vi "Vision 1.vi"(6 "Blue":cluster{"Lower value":i32, "Upper value":i32}={"Lower value"=0, "Upper value"=20}, 8 "Green":cluster{"Lower value":i32, "Upper value":i32}={"Lower value"=0, "Upper value"=20}, 10 "Red":cluster{"Lower value":i32, "Upper value":i32}={"Lower value"=0, "Upper value"=20}, 11 "RGB":T1) -> (0 "RGB":T1, 4 "Binary":T1)   [LabVIEW 2014]
uses:
  <vilib>/vision/Image Controls.llb/IMAQ Image.ctl
  <vilib>/vision/NI_Vision_Development_Module.lvlib
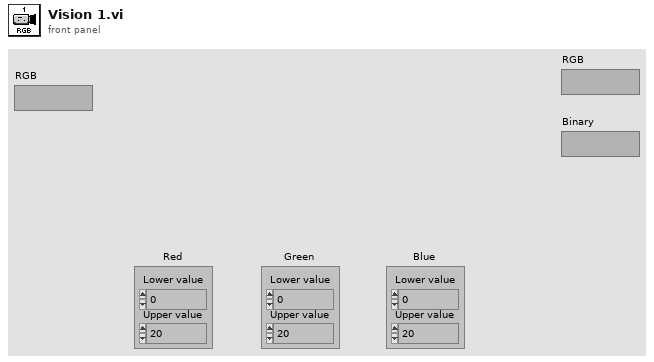
[diagram p1: front panel]
types:
  T1 = typedef "IMAQ Image.ctl" = refnum<image>
  T2 = typedef "Image Type" = u32
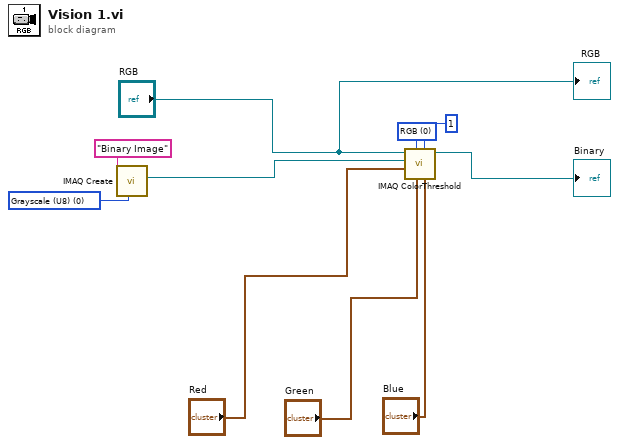
[diagram p0: block diagram]
diagram:
  w2 = T2 0 items=["Grayscale (U8)", "Grayscale (I16)", "Grayscale (SGL)", "Complex (CSG)", "RGB (U32)", "HSL (U32)", "RGB (U64)", "Grayscale (U16)"] ("Image Type")
  w7 = u16 0 items=["RGB", "HSL", "HSV", "HSI"] ("Color Mode")
  n1 = call "IMAQ Create"("Image Name"="Binary Image", "Image Type"=w2) -> ("New Image"=w1:T1)  [unwired: 3 in, 1 out]
  n2 = call "IMAQ ColorThreshold"("Blue or Luma or Val or Inten Range"="Blue", "Replace Value"=1, "Green or Sat Range"="Green", "Color Mode"=w7, "Red or Hue Range"="Red", "Image Dst"=w1, "Image Src"="RGB") -> ("Image Dst Out"=→"Binary":T1)  [unwired: 3 in, 1 out]
  "RGB" <- "RGB"
